vi "status.vi"(1 "VCI_CAN_STATUS":T1) -> ()   [LabVIEW 2013]
panel:
  out "Reserved":u32
  out "regTECounter":u8
  out "regRECounter":u8
  out "regEWLimit":u8
  out "regECCapture":u8
  out "regALCapture":u8
  out "regStatus":u8
  out "regMode":u8
  out "ErrInterrupt":u8
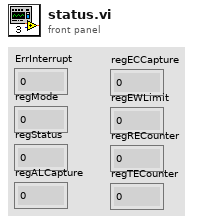
[diagram p1: front panel]
types:
  T1 = cluster{"ErrInterrupt":u8, "regMode":u8, "regStatus":u8, "regALCapture":u8, "regECCapture":u8, "regEWLimit":u8, "regRECounter":u8, "regTECounter":u8, "Reserved":u32}
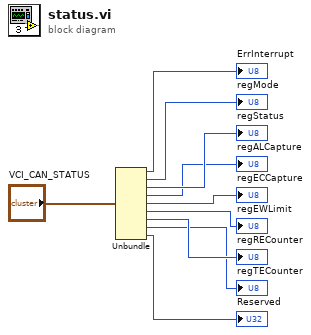
[diagram p0: block diagram]
diagram:
  n1 = Unbundle("VCI_CAN_STATUS") -> ("ErrInterrupt"=→"ErrInterrupt":u8, "regMode"=→"regMode":u8, "regStatus"=→"regStatus":u8, "regALCapture"=→"regALCapture":u8, "regECCapture"=→"regECCapture":u8, "regEWLimit"=→"regEWLimit":u8, "regRECounter"=→"regRECounter":u8, "regTECounter"=→"regTECounter":u8, "Reserved"=→"Reserved":u32)
